vi "DSF.Shared.Configuration.JSON.Write File.vi"(8 "error in (no error)":errorcluster, 9 "json string":string, 10 "path":path, 11 "JSON Configuration in":refnum<class "DSF.Shared.Configuration.JSON.lvclass">) -> (0 "error out":errorcluster, 3 "JSON Configuration out":refnum<class "DSF.Shared.Configuration.JSON.lvclass">)   [LabVIEW 2017, in "DSF.Shared.lvlib" / "DSF.Shared.Configuration.JSON.lvclass"]
uses:
  DSF.Shared.Configuration.JSON.lvclass
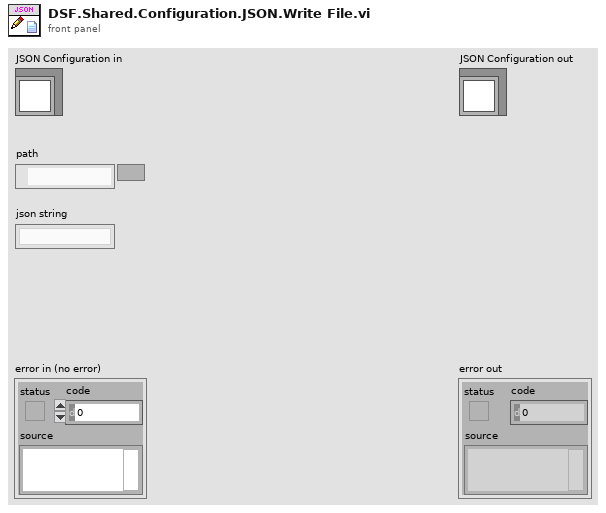
[diagram p1: front panel]
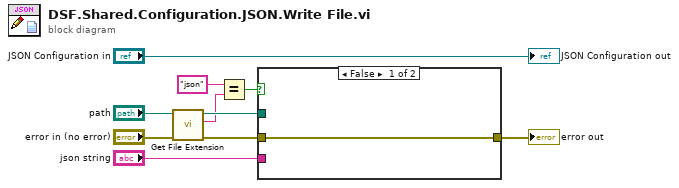
[diagram p0: block diagram]
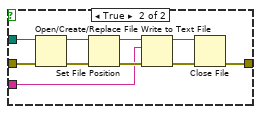
[diagram p2: hidden frame]
diagram:
  n1 = call <vilib>:"Get File Extension.vi"("error in (no error)"="error in (no error)", "file"="path") -> ("error out"=w6:errorcluster, "lowercase file extension"=w4:string, "dup file"=w5:path)  [unwired: 5 in, 2 out]
  n2 = Equal?(x="json", y=w4) -> (x = y?=w2:bool)
  n3 = case shown="False" w2 {
    tunnel: [w11 w19] -> w9
    tunnel: w6 -> [w11 w18]
    tunnel: w5 -> [_ w17]
    tunnel: "json string" -> [_ w12]
    frame False {
    }
    frame True {
      n4 = Open/Create/Replace File(file path (use dialog)=w17, error in=w18) -> (refnum out=w21:refnum<file>, error out=w20:errorcluster)  [unwired: 4 in, 1 out]
      n5 = Set File Position(refnum=w21, error in=w20) -> (refnum out=w16:refnum<file>, error out=w15:errorcluster)  [unwired: 2 in]
      n6 = Write to Text File(file (use dialog)=w16, text=w12, error in=w15) -> (refnum out=w14:refnum<file>, error out=w13:errorcluster)  [unwired: 1 in, 1 out]
      n7 = Close File(refnum=w14, error in=w13) -> (error out=w19:errorcluster)  [unwired: 1 out]
    }
  }
  "error out" <- w9
  "JSON Configuration out" <- "JSON Configuration in"
